vi "DrivePath.vi"() -> ()   [LabVIEW 2020]
uses:
  Dawgma Programming Library/Controls/PurePursuit/PathFileData.ctl
  Dawgma Programming Library/Controls/PurePursuit/RobotNeededPathData.ctl
  Framework/Robot Global Data.vi
panel:
  in  "NoWait":bool
  in  "Index":dbl
  in  "PathFileName":string
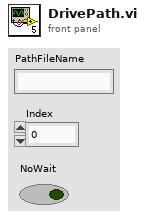
[diagram p1: front panel]
types:
  T1 = typedef "PathFileData.ctl" = cluster{"RobotNeeded":T2, "Meta":cluster{"Path (px)":cluster{i32, i32}[], "RobotWidth":dbl, "RobotLength":dbl, "CenterOfRotYOffset":dbl, "Roundedness":dbl, "StartingPositionPreset":u32, "PathName":string}}
  T2 = typedef "RobotNeededPathData.ctl" = cluster{"Path":cluster{dbl, dbl}[], "MaxVel":dbl, "MaxAccel":dbl, "Backwards?":bool, "PointSpacing":dbl, "LookaheadDist":dbl, "Speed/Curve":dbl, "SlowDistanceAtEnd":dbl, "SlowSpeed":dbl, "MaxDeAccel":dbl}
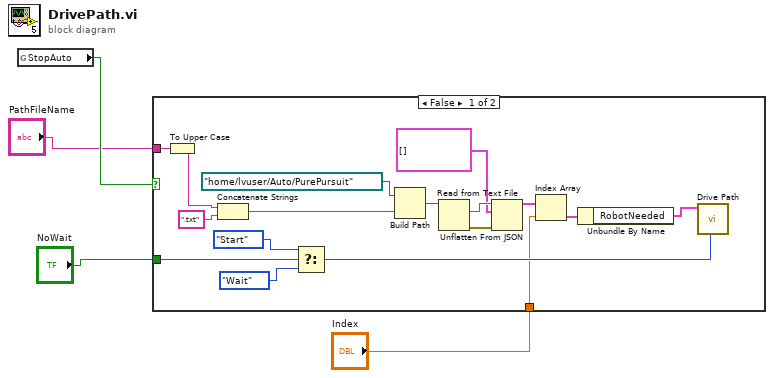
[diagram p0: block diagram]
diagram:
  n1 = global read "Robot Global Data.vi" "StopAuto"() -> (w4:bool)
  n2 = case shown="False" w4 {
    tunnel: "NoWait" -> [w9 _]
    tunnel: "Index" -> [w7 _]
    tunnel: "PathFileName" -> [w6 _]
    frame False {
      n3 = To Upper Case(1:w6) -> (0:w5:string)
      n4 = Concatenate Strings(w5, ".txt" ("string")) -> (w20:string)
      n5 = Select(t=enum16{"Start", "Wait"}."Start" ("Synchronication"), s=w9, f=enum16{"Start", "Wait"}."Wait" ("Synchronication")) -> (s? t:f=w8:enum16{"Start", "Wait"})
      n6 = Build Path(base path=path "/home/lvuser/Auto/PurePursuit", name or relative path=w20) -> (appended path=w18:path)
      n7 = Read from Text File(file (use dialog)=w18) -> (text=w16:string, error out=w17:errorcluster)  [unwired: 3 in, 2 out]
      n8 = Unflatten From JSON(JSON string=w16, type and defaults=T1[] [], error in (no error)=w17) -> (value=w14:T1[])  [unwired: 4 in, 1 out]
      n9 = Index Array(array=w14, index=w7) -> (element=w13:T1)
      n10 = Unbundle By Name(w13) -> ("RobotNeeded"=w12:T2)
      n11 = call "Drive Path.vi"("Synchronication"=w8, "RobotNeededPathData"=w12) -> ()  [unwired: 9 in, 1 out]
    }
    frame True {
    }
  }
